vi "Diagnostic.vi"(7 "Unit Address (1)":i16=1, 8 "error in (no error)":errorcluster {"code" format="%.0x"}, 10 "Item To Read (0: Input 1 Type)":u16(ring) items=["Input 1 Type", "Input 2 Type", "Input 3 Type", "Output 1A Type", "Output 1B Type", "Output 2A Type", "Output 2B Type", "Retransmit 1", "Retransmit 2", "CJC1 Temp", "CJC2 Temp", "Line Frequency"], 11 "VISA resource name":refnum<visa-resource-name>) -> (0 "error out":errorcluster {"code" format="%.0x"}, 2 "Value":dbl format="%.2f", 3 "VISA resource name out":refnum<visa-resource-name>)   [LabVIEW 2010]
doc: "This VI returns base instrument informations."
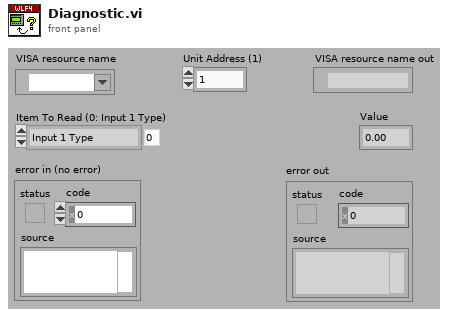
[diagram p1: front panel]
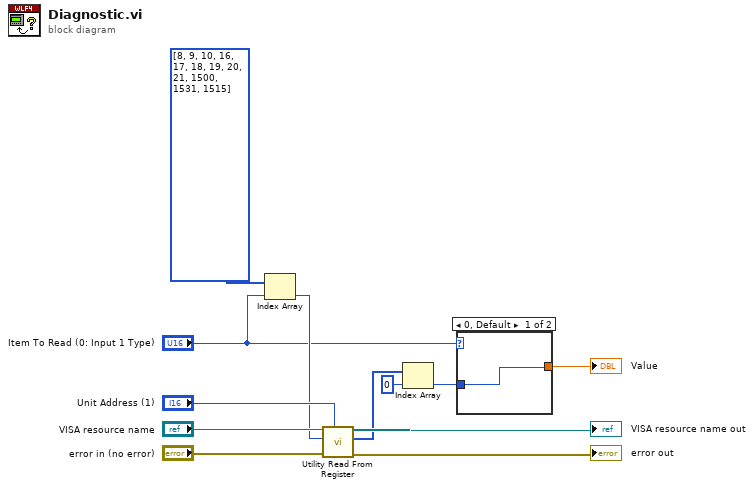
[diagram p0: block diagram]
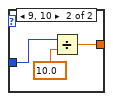
[diagram p2: hidden frame]
diagram:
  n1 = Index Array(array=i32[] [8, 9, 10, 16, 17, 18, 19, 20, 21, 1500, 1531, 1515], index="Item To Read (0: Input 1 Type)") -> (element=w6:i32)
  n2 = call "Utility Read From Register.vi"("Unit Address (1)"="Unit Address (1)", "error in (no error)"="error in (no error)", "Register Address (0)"=w6, "VISA resource name"="VISA resource name") -> ("error out"=→"error out":errorcluster, "Data"=w2:i16[], "VISA resource name out"=→"VISA resource name out":refnum<visa-resource-name>)  [unwired: 5 in]
  n3 = Index Array(array=w2, index=0) -> (element=w1:i16)
  n4 = case shown="0, Default" "Item To Read (0: Input 1 Type)" {
    tunnel: [w13 w15] -> w5
    tunnel: w1 -> [w13 w14]
    frame 0, Default {
    }
    frame 9, 10 {
      n5 = Divide(x=w14, y=10.0) -> (x/y=w15:dbl)
    }
  }
  "Value" <- w5
